vi "configuration.vi"(4 "force_read?":bool, 6 "custom_file":path, 7 "command":T1=enum."read_config", 8 "error in (no error)":errorcluster, 10 "project_file":path, 11 "config in":T2) -> (0 "error out":errorcluster, 3 "config out":T2)   [LabVIEW 2015, in "lv-builder-l3.lvlib"]
doc: "This VI is able to read/write configuration from all the associated modules defined in the master data cluster. It also acts as a functional global/data store in the event that no data has changed since the last write. It will self-initialize and well set an internal flag in the event an error is encountered when reading. If no command is provided, it will default to the read command."
uses:
  lv-builder-l3.lvlib
  public/_controls/configuration.ctl
  _controls/configuration_command.ctl
  <userlib>/antonio-alexander/lv-build/lv-build/lv-build.lvlib
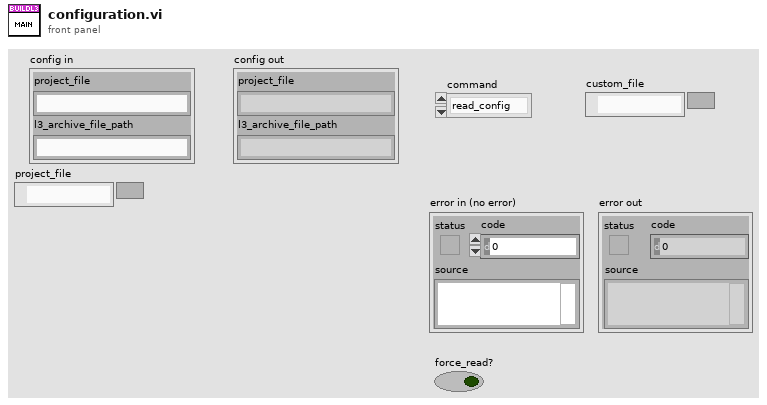
[diagram p1: front panel]
types:
  T1 = typedef "lv-builder-l3.lvlib/configuration_command.ctl" = enum16{"<config_command>", "read_config", "write_config", "<null>"}
  T2 = typedef "lv-builder-l3.lvlib/configuration.ctl" = cluster{"project_file":string, "l3_archive_file_path":string}
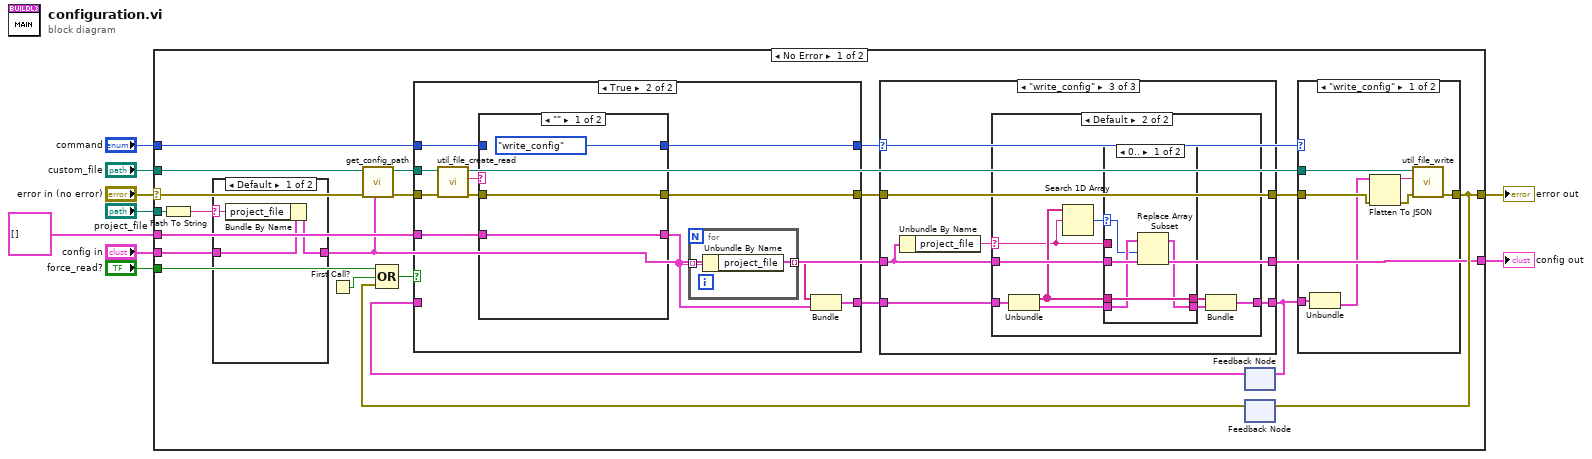
[diagram p0: block diagram]
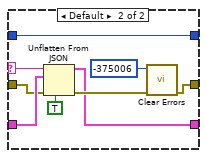
[diagram p4: hidden frame]
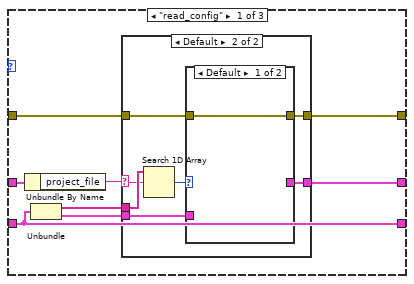
[diagram p5: hidden frame]
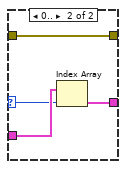
[diagram p7: hidden frame]
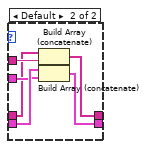
[diagram p10: hidden frame]
diagram:
  n1 = case shown="No Error" "error in (no error)" {
    selector: "error in (no error)" -> [w15 w122]
    tunnel: "command" -> [w24 _]
    tunnel: [w31 w122] -> w5
    tunnel: "config in" -> [w11 _]
    tunnel: "custom_file" -> [w17 _]
    tunnel: [w18 _] -> w4
    tunnel: "force_read?" -> [w28 _]
    tunnel: T2[] [] ("default") -> [w25 _]
    tunnel: "project_file" -> [w13 _]
    frame No Error {
      n2 = Path To String(path=w13) -> (string=w12:string)
      n3 = case shown="Default" w12 {
        selector: w12 -> [w32 _]
        tunnel: w11 -> [w34 w35]
        tunnel: [w33 w35] -> w10
        frame Default {
          n4 = Bundle By Name(cluster=w34, "project_file"=w32) -> (w33:T2)
        }
        frame "" {
        }
      }
      n5 = First Call?() -> (First Call?: T/F=w29:bool)
      n6 = call "get_config_path.vi"("configuration"=w10, "error in (no error)"=w15, "custom_file"=w17) -> ("error out"=w14:errorcluster, "config_path"=w16:path)  [unwired: 7 in]
      n7 = feedback #1() -> (w26:cluster{string[], "default":T2[]})  [unwired: 1 in]
      n8 = feedback #2() -> (w30:errorcluster)  [unwired: 1 in]
      n9 = Compound Arithmetic op=OR(w28, w29, w30) -> (w27:bool)
      n10 = case shown="True" w27 {
        tunnel: w26 -> [w38 _]
        tunnel: w14 -> [w37 w47]
        tunnel: w16 -> [_ w48]
        tunnel: [w37 w45] -> w22
        tunnel: w25 -> [_ w49]
        tunnel: w24 -> [w36 w44]
        tunnel: [w36 w43] -> w23
        tunnel: [w38 w39] -> w19
        frame False {
        }
        frame True {
          n11 = call <userlib>:"util_file_create_read.vi"("error in (no error)"=w47, "config_path"=w48) -> ("error out"=w46:errorcluster, "string"=w42:string)  [unwired: 8 in]
          n12 = case shown="\"\"" w42 {
            selector: w42 -> [_ w59]
            tunnel: w49 -> [w53 w62]
            tunnel: [w53 w61] -> w40
            tunnel: w46 -> [w54 w60]
            tunnel: [w54 w55] -> w45
            tunnel: w44 -> [_ w58]
            tunnel: [configuration_command."write_config" ("command") w58] -> w43
            frame "" {
            }
            frame Default {
              n13 = Unflatten From JSON(JSON string=w59, type and defaults=w62, default null elements? (F)=TRUE, error in (no error)=w60) -> (value=w61:T2[], error out=w63:errorcluster)  [unwired: 3 in]
              n14 = call <vilib>:"Clear Errors.vi"("error in (no error)"=w63, "specific error code to clear (0: all)"=-375006) -> ("error out"=w55:errorcluster)  [unwired: 4 in, 1 out]
            }
          }
          n15 = for {
            tunnel: w40 -> [w51] mode=indexing
            tunnel: [w50] -> w41 mode=indexing
            n16 = Unbundle By Name(w51) -> ("project_file"=w50:string)
          }
          n17 = Bundle(w41, "default"=w40) -> (w39:cluster{string[], "default":T2[]})  [unwired: 1 in]
        }
      }
      n18 = case shown="\"write_config\"" w23 {
        tunnel: w10 -> [w67 w87 w89]
        tunnel: [w71 w86 w92] -> w20
        tunnel: w19 -> [w71 w86 w90]
        tunnel: [w66 w87 w89] -> w18
        tunnel: w22 -> [w65 w85 w88]
        tunnel: [w64 w85 w88] -> w21
        frame "read_config" {
          n19 = Unbundle By Name(w67) -> ("project_file"=w68:string)
          n20 = Unbundle(w71) -> (w70:string[], "default"=w69:T2[])
          n21 = case shown="Default" w68 {
            selector: w68 -> [_ w76]
            tunnel: w70 -> [_ w79]
            tunnel: w69 -> [_ w78]
            tunnel: [_ w75] -> w66
            tunnel: w65 -> [w72 w74]
            tunnel: [w72 w73] -> w64
            frame "" {
            }
            frame Default {
              n22 = Search 1D Array(1D array=w79, element=w76) -> (index of element=w77:i32)  [unwired: 1 in]
              n23 = case shown="Default" w77 {
                selector: w77 -> [_ w83]
                tunnel: w78 -> [_ w84]
                tunnel: [_ w82] -> w75
                tunnel: w74 -> [w80 w81]
                tunnel: [w80 w81] -> w73
                frame Default {
                }
                frame 0.. {
                  n24 = Index Array(array=w84, index=w83) -> (element=w82:T2)
                }
              }
            }
          }
        }
        frame Default {
        }
        frame "write_config" {
          n25 = Unbundle By Name(w89) -> ("project_file"=w91:string)
          n26 = case shown="Default" w91 {
            selector: w91 -> [_ w94]
            tunnel: [w93 w100] -> w92
            tunnel: w89 -> [_ w98]
            tunnel: w90 -> [w93 w96]
            frame "" {
            }
            frame Default {
              n27 = Unbundle(w96) -> (w95:string[], "default"=w97:T2[])
              n28 = Search 1D Array(1D array=w95, element=w94) -> (index of element=w102:i32)  [unwired: 1 in]
              n29 = case shown="0.." w102 {
                selector: w102 -> [w103 _]
                tunnel: w97 -> [w106 w112]
                tunnel: [w105 w110] -> w101
                tunnel: w95 -> [w107 w108]
                tunnel: [w107 w109] -> w99
                tunnel: w98 -> [w104 w111]
                tunnel: w94 -> [_ w113]
                frame 0.. {
                  n30 = Replace Array Subset(array=w106, new element=w104, index=w103) -> (w105:T2[])
                }
                frame Default {
                  n31 = Build Array (concatenate)(w108, w113) -> (w109:string[])
                  n32 = Build Array (concatenate)(w112, w111) -> (w110:T2[])
                }
              }
              n33 = Bundle(w99, "default"=w101) -> (w100:cluster{string[], "default":T2[]})  [unwired: 1 in]
            }
          }
        }
      }
      n34 = feedback-in #1(w20) -> ()
      n35 = case shown="\"write_config\"" w23 {
        tunnel: w20 -> [w117 _]
        tunnel: w21 -> [w118 w121]
        tunnel: [w115 w121] -> w31
        tunnel: w16 -> [w116 _]
        frame "write_config" {
          n36 = Unbundle(w117) -> ("default"=w114:T2[])  [unwired: 1 out]
          n37 = Flatten To JSON(anything=w114, error in (no error)=w118) -> (JSON string=w120:string, 11:w119:errorcluster)  [unwired: 1 in]
          n38 = call <userlib>:"util_file_write.vi"("error in (no error)"=w119, "string"=w120, "config_path"=w116) -> ("error out"=w115:errorcluster)  [unwired: 8 in]
        }
        frame Default {
        }
      }
      n39 = feedback-in #2(w31) -> ()
    }
    frame Error {
      # "If an error is wired in, be sure to skip over functionality to preserve the original error"
    }
  }
  "config out" <- w4
  "error out" <- w5
